vi "Paragraph_SetStyleName.vi"(8 "error in":errorcluster, 10 "StyleName":string, 11 "Paragraph":refnum<k24>) -> (0 "error out":errorcluster, 3 "Paragraph dup":refnum<k24>)   [LabVIEW 2009]
uses:
  C:/Projets/LAVAG/OpenOfficeRGT/AODL/DLLs/AODL.dll
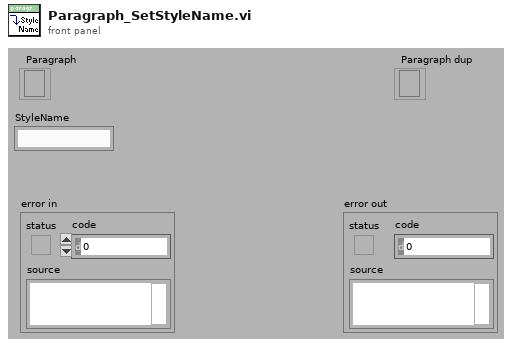
[diagram p1: front panel]
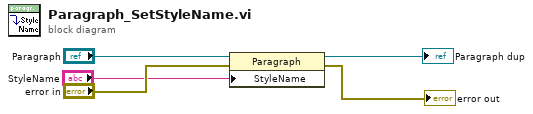
[diagram p0: block diagram]
diagram:
  n1 = property class="Paragraph"(reference="Paragraph", error in="error in", "StyleName"="StyleName") -> (reference out=→"Paragraph dup":refnum<k24>, error out=→"error out":errorcluster)
